vi "Compute Possible Connections.vi"(8 "error in (no error)":errorcluster, 11 "Item Ref in":T2 format="%.0x") -> (0 "error out":errorcluster, 2 "Possible Connections":T1[](array[typedef]), 3 "Item Ref out":T2 format="%.0x")   [LabVIEW 2017, in "SLSC Switch Scripting.lvlib"]
uses:
  SLSC Switch Scripting.lvlib
  <vilib>/NI Veristand/Custom Device API/Custom Device Item Ref.ctl
  Shared/Routing and Faulting Hardware API/Types/Possible Connections for Endpoint.ctl
  <vilib>/SLSC_Switch/Initialize with Topology (Simulate).vi
  <vilib>/SLSC_Switch/SLSC Switch.lvlib
  Shared/Routing and Faulting Hardware API/Routing and Faulting Hardware API.lvlib
  <vilib>/NI Veristand/Custom Device API/Custom Device API.lvlib
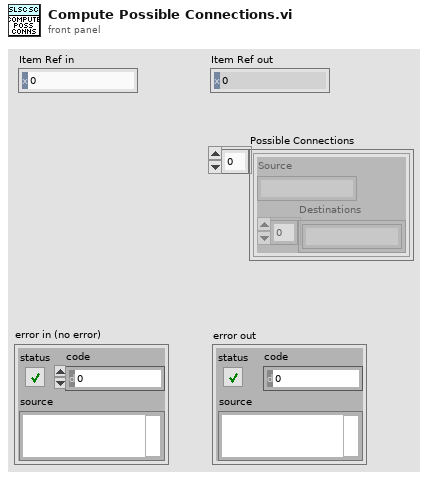
[diagram p1: front panel]
types:
  T1 = typedef "Routing and Faulting Hardware API.lvlib/Possible Connections for Endpoint.ctl" = cluster{"Source":string, "Destinations":string[]}
  T2 = typedef "Custom Device API.lvlib/Custom Device Item Ref.ctl" = u64
  T3 = typedef "nislscslSession.ctl" = refnum<k20>
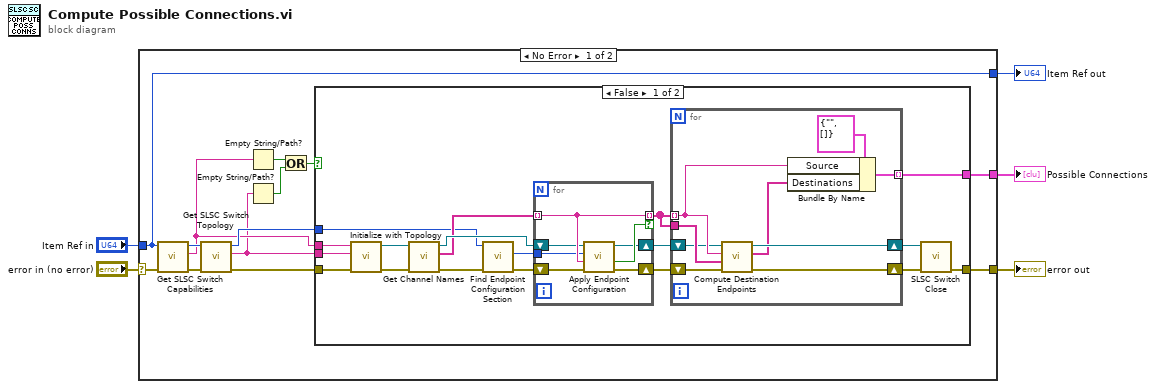
[diagram p0: block diagram]
diagram:
  n1 = case shown="No Error" "error in (no error)" {
    selector: "error in (no error)" -> [w14 w55]
    tunnel: [w18 w55] -> w5
    tunnel: "Item Ref in" -> [w8 w54]
    tunnel: [w8 w54] -> w3
    tunnel: [w12 _] -> w1
    frame No Error {
      n2 = call "Get SLSC Switch Capabilities.vi"("error in (no error)"=w14, "SLSC Switch Custom Device Ref in"=w8) -> ("error out"=w17:errorcluster, "Capabilities"=w11:string, "SLSC Switch Custom Device Ref out"=w16:T2)  [unwired: 7 in]
      n3 = call "Get SLSC Switch Topology.vi"("error in (no error)"=w17, "SLSC Switch Custom Device Ref in"=w16) -> ("error out"=w13:errorcluster, "Topology"=w10:string, "SLSC Switch Custom Device Ref out"=w15:T2)  [unwired: 7 in]
      n4 = Empty String/Path?(string/path=w11) -> (empty?=w6:bool)
      n5 = Empty String/Path?(string/path=w10) -> (empty?=w7:bool)
      n6 = Or(x=w6, y=w7) -> (x .or. y?=w9:bool)
      n7 = case shown="False" w9 {
        tunnel: [w27 w53] -> w18
        tunnel: w11 -> [w26 _]
        tunnel: w10 -> [w25 _]
        tunnel: w15 -> [w20 _]
        tunnel: w13 -> [w24 w53]
        tunnel: [w23 _] -> w12
        frame False {
          n8 = call-poly <vilib>:"Initialize with Topology.vi"("error in (no error)"=w24, "topology"=w25, "switches json"=w26) -> ("error out"=w32:errorcluster, "session out"=w35:T3)  [unwired: 7 in]
          n9 = call <vilib>:"Get Channel Names.vi"("error in (no error)"=w32, "session in"=w35) -> ("error out"=w22:errorcluster, "channel names"=w33:string[], "session out"=w34:T3)  [unwired: 7 in]
          n10 = call "Find Endpoint Configuration Section.vi"("error in (no error)"=w22, "SLSC Switch Custom Device Ref in"=w20) -> ("error out"=w21:errorcluster, "Endpoint Config Section Ref"=w19:T2)  [unwired: 7 in, 1 out]
          n11 = for {
            tunnel: [w40] -> w36 mode=indexing if=w43
            tunnel: w33 -> [w40] mode=indexing
            tunnel: w19 -> [w38]
            shift-right: [w41] -> w31
            shift-left: w21 -> [w42]
            shift-right: [w37] -> w30
            shift-left: w34 -> [w39]
            n12 = call "Apply Endpoint Configuration.vi"("error in (no error)"=w42, "Endpoint"=w40, "Endpoint Config Section Ref in"=w38, "Refnum in"=w39) -> ("error out"=w41:errorcluster, "Endpoint Addressable?"=w43:bool, "Refnum out"=w37:T3)  [unwired: 4 in, 1 out]
          }
          n13 = for {
            tunnel: w36 -> [w47] mode=indexing
            tunnel: w36 -> [w52]
            shift-right: [w50] -> w29
            shift-left: w31 -> [w51]
            shift-right: [w49] -> w28
            shift-left: w30 -> [w44]
            tunnel: [w45] -> w23 mode=indexing
            n14 = call "Compute Destination Endpoints.vi"("error in (no error)"=w51, "Endpoints"=w52, "Source Endpoint"=w47, "Refnum in"=w44) -> ("error out"=w50:errorcluster, "Possible Destination Endpoints"=w46:string[], "Refnum out"=w49:T3)  [unwired: 5 in]
            n15 = Bundle By Name(cluster=T1 {"Source"="", "Destinations"=[]} ("Possible Connections for Endpoint"), "Source"=w47, "Destinations"=w46) -> (w45:T1)
          }
          n16 = call "SLSC Switch Close.vi"("error in (no error)"=w29, "session in"=w28) -> ("error out"=w27:errorcluster)  [unwired: 9 in]
        }
        frame True {
        }
      }
    }
    frame Error {
    }
  }
  "error out" <- w5
  "Item Ref out" <- w3
  "Possible Connections" <- w1
